vi "Bsweep_VgDep.vi"(5 "Time Stamp":timestamp, 6 "Play Button":bool, 7 "Rate w/o measure, T/min":dbl=0.5 min=0.0 max=1.0 step=0.01 format="%.4f", 9 "Sweep rate, T/min":dbl=0.2 min=0.0 max=1.0 step=0.01 format="%.4f", 10 "B2 (T)":dbl=0.5 min=-4.0 max=4.0 step=0.1 format="%.4f", 11 "B1 (T)":dbl=-0.5 min=-4.0 max=4.0 step=0.1 format="%.4f") -> ()   [LabVIEW 2015]
uses:
  <vilib>/Utility/file.llb/Read From Spreadsheet File (DBL).vi
panel:
  in  "Custom Folder":string
  in  "Hysteresis":bool
  out "VgArray":dbl[](array[numeric])
  in  "Step (V)":dbl=3.0 min=-4.0 max=4.0 step=0.1 format="%.3f"
  in  "Final Vg (V)":dbl=3.0 min=-4.0 max=4.0 step=0.1 format="%.3f"
  in  "Initial Vg (V)":dbl=-3.0 min=-4.0 max=4.0 step=0.1 format="%.3f"
  out "Experiment ends at:":string
  out "Hours":dbl format="%.1f"
  out "Estimated time of experiment:":i16
  in  "Ramp rate (V/min)":dbl=30.0
  in  "Quick Mode":bool=TRUE
  out "Numeric":dbl
  out "Communication":string
  out "ArraySens":i8[](array[numeric])
  out "ArrayOsc":dbl[](array[numeric])
  out "# of configurations":i8
  out "Large Array":bool[][][](array[boolean])
  out "Contact configuration file (*.conf)":path
  # "Set gate voltages at which B-sweeps\nare made"
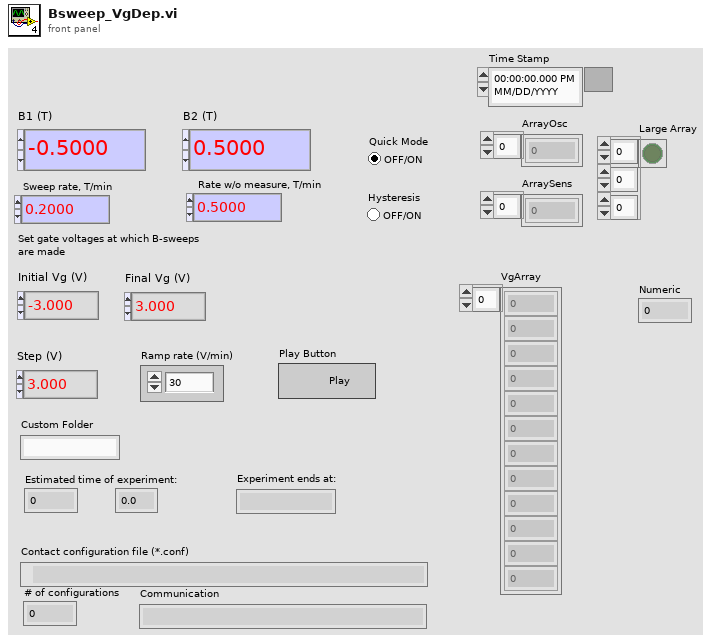
[diagram p1: front panel]
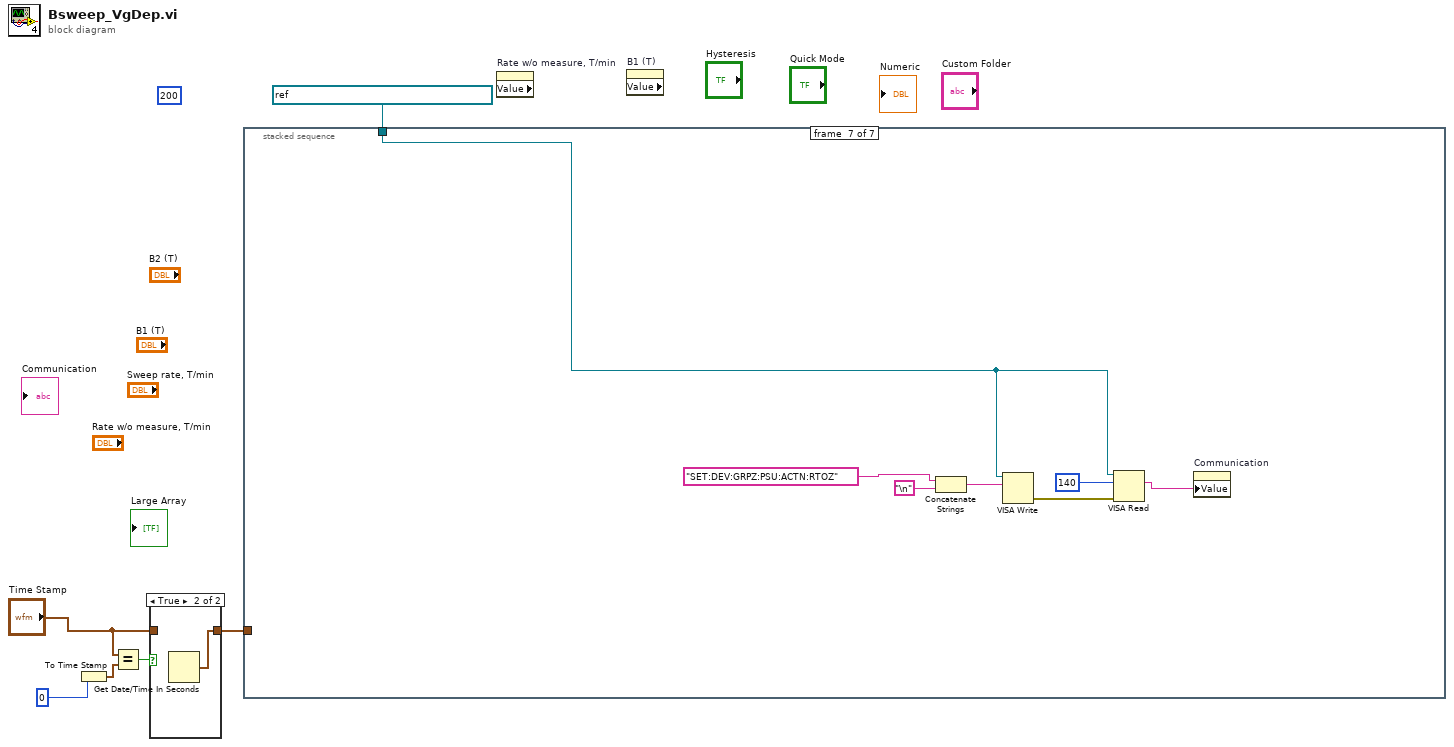
[diagram p0: block diagram]
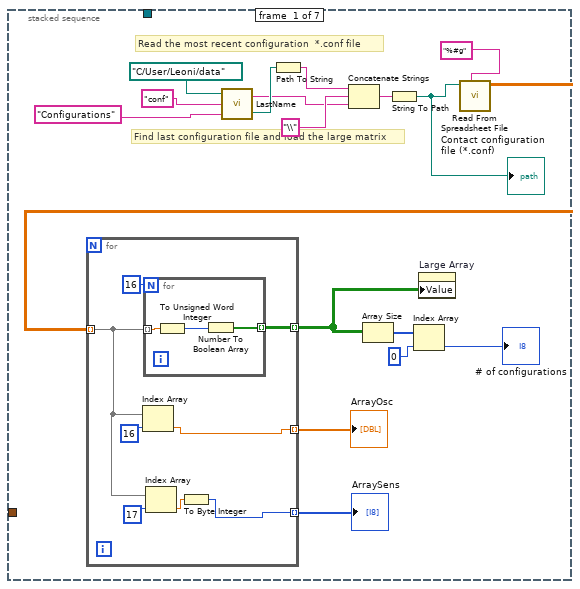
[diagram p3: hidden frame]
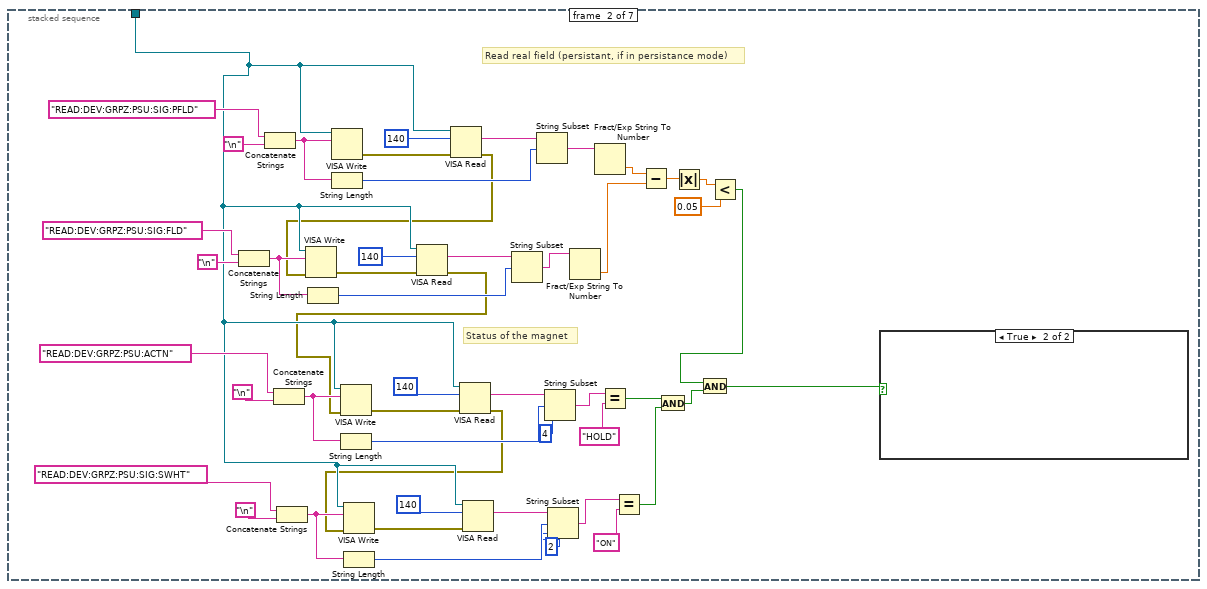
[diagram p4: hidden frame]
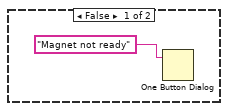
[diagram p5: hidden frame]
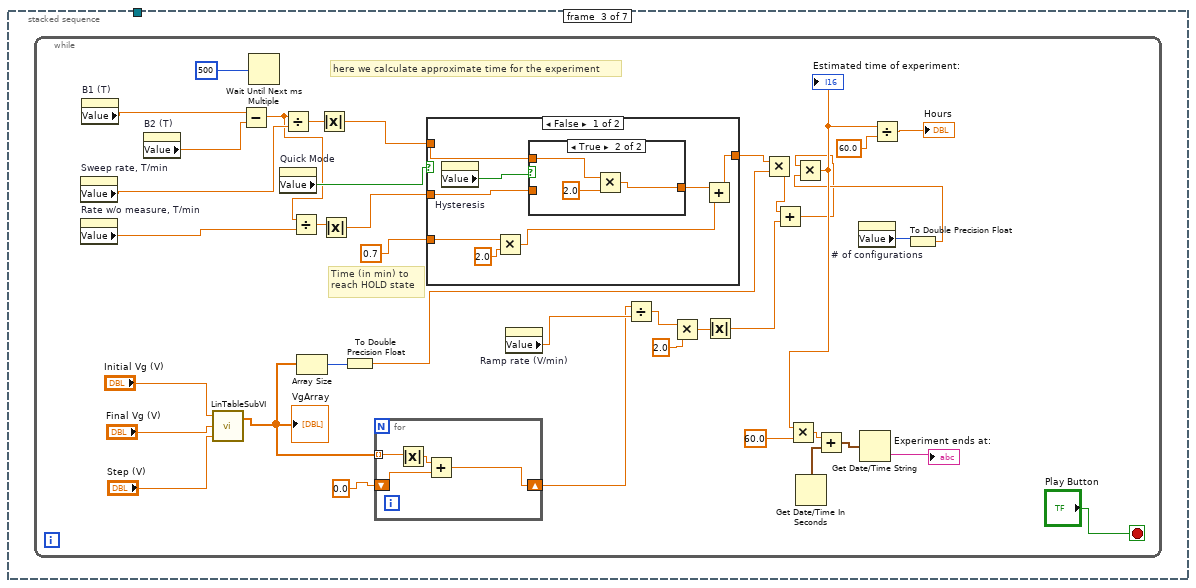
[diagram p6: hidden frame]
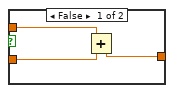
[diagram p7: hidden frame]
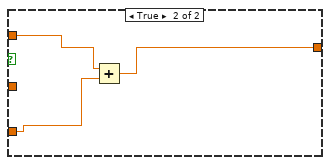
[diagram p8: hidden frame]
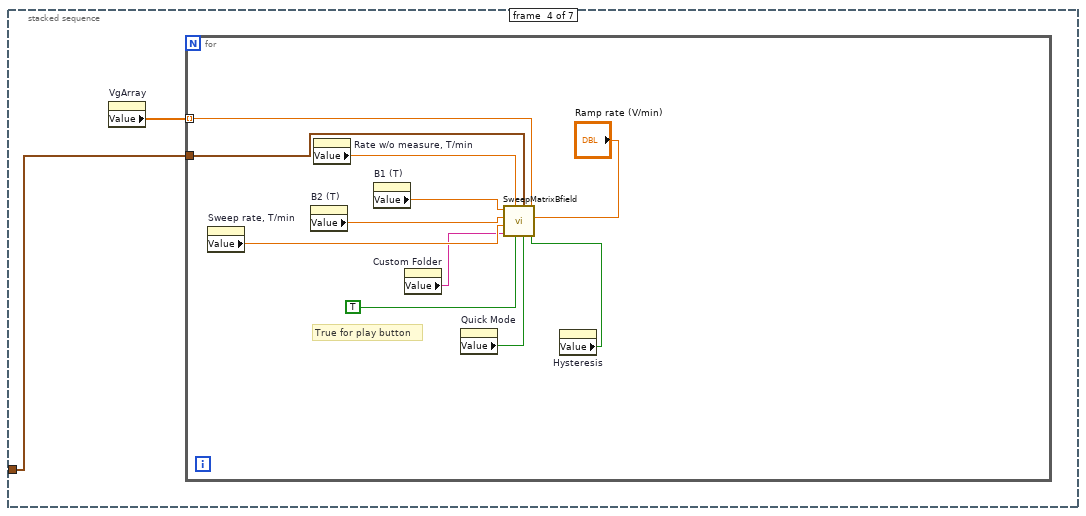
[diagram p9: hidden frame]
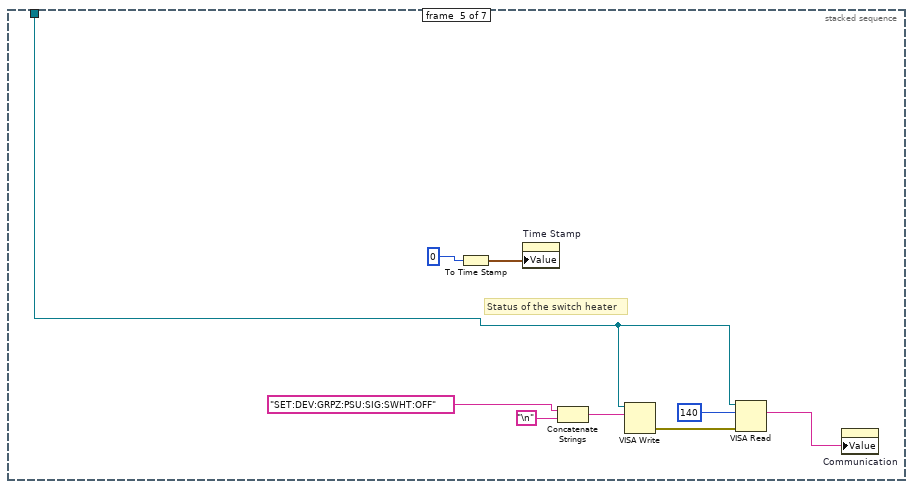
[diagram p10: hidden frame]
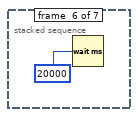
[diagram p11: hidden frame]
diagram:
  (unwired) 200
  n1 = To Time Stamp(1:0) -> (0:w4:timestamp)
  n2 = Equal?(x="Time Stamp", y=w4) -> (x = y?=w3:bool)
  n3 = case shown="True" w3 {
    tunnel: "Time Stamp" -> [w7 _]
    tunnel: [w7 w8] -> w1
    frame False {
    }
    frame True {
      n4 = Get Date/Time In Seconds() -> (seconds since 1Jan1904=w8:timestamp)
    }
  }
  n5 = stacked-sequence {
    tunnel: refnum<visa-resource-name> "TCPIP0::192.168.128.3::7020::SOCKET" ("VISA resource name") -> [_ w40 _ _ w162 _ w172]
    tunnel: w1 -> [_ _ _ w148 _ _ _]
    frame #0 {
      # "Read the most recent configuration  *.conf file"
      # "Find last configuration file and load the large matrix"
      n6 = call "LastName.vi"("Custom Folder"="Configurations", "Extention"="conf", "User Data Folder"=path "C:/User/Leoni/data") -> ("created path"=w21:path, "String"=w20:string)
      n7 = Path To String(path=w21) -> (string=w25:string)
      n8 = Concatenate Strings(w25, "\\", w20) -> (w23:string)
      n9 = String To Path(string=w23) -> (path=w11:path)
      "Contact configuration file (*.conf)" <- w11
      n10 = call-poly <vilib>:"Read From Spreadsheet File.vi"("format (%.3f)"="%#g", "file path (dialog if empty)"=w11) -> ("all rows"=w16:dbl[][])  [unwired: 5 in, 4 out]
      n11 = for {
        tunnel: w16 -> [w29] mode=indexing
        tunnel: [w33] -> w13 mode=indexing
        tunnel: [w28] -> w10 mode=indexing
        tunnel: [w27] -> w9 mode=indexing
        n12 = Index Array(array=w29, index=16) -> (element=w28:dbl)
        n13 = for {
          N: 16 -> [_]
          tunnel: w29 -> [w36] mode=indexing
          tunnel: [w34] -> w33 mode=indexing
          n14 = To Unsigned Word Integer(number=w36) -> (unsigned 16bit integer=w35:u16)
          n15 = Number To Boolean Array(number=w35) -> (Boolean array=w34:bool[])
        }
        n16 = Index Array(array=w29, index=17) -> (element=w30:dbl)
        n17 = To Byte Integer(number=w30) -> (8bit integer=w27:i8)
      }
      "ArrayOsc" <- w10
      "ArraySens" <- w9
      n18 = Array Size(array=w13) -> (size(s)=w15:i32[])
      n19 = Index Array(array=w15, index=0) -> (element=→"# of configurations":i32)
      n20 = property on="Large Array" class="Arr (strict)"("Value"=w13) -> ()  [unwired: 2 in, 2 out]
    }
    frame #1 {
      # "Status of the magnet"
      # "Read real field (persistant, if in persistance mode)"
      n21 = Concatenate Strings("READ:DEV:GRPZ:PSU:SIG:FLD" ("string"), "\n") -> (w74:string)
      n22 = Concatenate Strings("READ:DEV:GRPZ:PSU:SIG:PFLD" ("string"), "\n") -> (w80:string)
      n23 = Concatenate Strings("READ:DEV:GRPZ:PSU:ACTN" ("string"), "\n") -> (w59:string)
      n24 = Concatenate Strings("READ:DEV:GRPZ:PSU:SIG:SWHT" ("string"), "\n") -> (w49:string)
      n25 = String Length(string=w74) -> (length=w72:i32)
      n26 = VISA Write(VISA resource name=w40, write buffer=w80) -> (error out=w86:errorcluster)  [unwired: 1 in, 2 out]
      n27 = String Length(string=w80) -> (length=w81:i32)
      n28 = String Length(string=w59) -> (length=w60:i32)
      n29 = String Length(string=w49) -> (length=w50:i32)
      n30 = VISA Read(VISA resource name=w40, byte count=140, error in (no error)=w86) -> (read buffer=w82:string, error out=w39:errorcluster)  [unwired: 2 out]
      n31 = VISA Write(VISA resource name=w40, write buffer=w74, error in (no error)=w39) -> (error out=w78:errorcluster)  [unwired: 2 out]
      n32 = VISA Read(VISA resource name=w40, byte count=140, error in (no error)=w78) -> (read buffer=w73:string, error out=w38:errorcluster)  [unwired: 2 out]
      n33 = VISA Write(VISA resource name=w40, write buffer=w59, error in (no error)=w38) -> (error out=w65:errorcluster)  [unwired: 2 out]
      n34 = VISA Read(VISA resource name=w40, byte count=140, error in (no error)=w65) -> (read buffer=w61:string, error out=w37:errorcluster)  [unwired: 2 out]
      n35 = VISA Write(VISA resource name=w40, write buffer=w49, error in (no error)=w37) -> (error out=w55:errorcluster)  [unwired: 2 out]
      n36 = VISA Read(VISA resource name=w40, byte count=140, error in (no error)=w55) -> (read buffer=w51:string)  [unwired: 3 out]
      n37 = String Subset(string=w73, offset (0)=w72) -> (substring=w71:string)  [unwired: 1 in]
      n38 = String Subset(string=w82, offset (0)=w81) -> (substring=w79:string)  [unwired: 1 in]
      n39 = String Subset(string=w61, offset (0)=w60, length (rest)=4) -> (substring=w57:string)
      n40 = String Subset(string=w51, offset (0)=w50, length (rest)=2) -> (substring=w46:string)
      n41 = Fract/Exp String To Number(string=w71) -> (number=w69:dbl)  [unwired: 3 in, 1 out]
      n42 = Fract/Exp String To Number(string=w79) -> (number=w70:dbl)  [unwired: 3 in, 1 out]
      n43 = Equal?(x=w57, y="HOLD") -> (x = y?=w45:bool)
      n44 = Equal?(x=w46, y="ON") -> (x = y?=w44:bool)
      n45 = Subtract(x=w70, y=w69) -> (x-y=w68:dbl)
      n46 = And(x=w45, y=w44) -> (x .and. y?=w43:bool)
      n47 = Absolute Value(x=w68) -> (abs(x)=w67:dbl)
      n48 = Less?(x=w67, y=0.05) -> (x < y?=w42:bool)
      n49 = And(x=w42, y=w43) -> (x .and. y?=w41:bool)
      n50 = case shown="True" w41 {
        frame False {
          n51 = One Button Dialog(message="Magnet not ready") -> ()  [unwired: 1 in, 1 out]
        }
        frame True {
        }
      }
    }
    frame #2 {
      n52 = while {
        stop <- "Play Button" stop-if-true
        # "Time (in min) to\nreach HOLD state"
        # "here we calculate approximate time for the experiment"
        n53 = property on="Sweep rate, T/min" class="DigNum (strict)"() -> ("Value"=w112:dbl)  [unwired: 2 in, 2 out]
        n54 = property on="Rate w/o measure, T/min" class="DigNum (strict)"() -> ("Value"=w111:dbl)  [unwired: 2 in, 2 out]
        n55 = property on="B1 (T)" class="DigNum (strict)"() -> ("Value"=w114:dbl)  [unwired: 2 in, 2 out]
        n56 = property on="B2 (T)" class="DigNum (strict)"() -> ("Value"=w113:dbl)  [unwired: 2 in, 2 out]
        n57 = call "LinTableSubVI.vi"("Step"="Step (V)", "Final"="Final Vg (V)", "Initial"="Initial Vg (V)") -> ("Array"=w93:dbl[])  [unwired: 1 in]
        "VgArray" <- w93
        n58 = Subtract(x=w114, y=w113) -> (x-y=w109:dbl)
        n59 = Wait Until Next ms Multiple(millisecond multiple=500) -> ()  [unwired: 1 out]
        n60 = property on="Quick Mode" class="Bool (strict)"() -> ("Value"=w110:bool)  [unwired: 2 in, 2 out]
        n61 = Divide(x=w109, y=w112) -> (x/y=w125:dbl)
        n62 = Divide(x=w109, y=w111) -> (x/y=w100:dbl)
        n63 = Array Size(array=w93) -> (size(s)=w92:i32)
        n64 = Absolute Value(x=w125) -> (abs(x)=w115:dbl)
        n65 = Absolute Value(x=w100) -> (abs(x)=w99:dbl)
        n66 = To Double Precision Float(number=w92) -> (double precision float=w91:dbl)
        n67 = for {
          tunnel: w93 -> [w130] mode=indexing
          shift-right: [w127] -> w94
          shift-left: 0.0 -> [w128]
          n68 = Absolute Value(x=w130) -> (abs(x)=w129:dbl)
          n69 = Add(x=w129, y=w128) -> (x+y=w127:dbl)
        }
        n70 = case shown="False" w110 {
          tunnel: [w132 w145] -> w101
          tunnel: w99 -> [w138 _]
          tunnel: w115 -> [w137 w147]
          tunnel: 0.7 -> [w135 w146]
          frame False {
            n71 = property on="Hysteresis" class="Bool (strict)"() -> ("Value"=w131:bool)  [unwired: 2 in, 2 out]
            n72 = Multiply(x=w135, y=2.0) -> (x*y=w134:dbl)
            n73 = case shown="True" w131 {
              tunnel: w138 -> [w141 _]
              tunnel: w137 -> [w140 w143]
              tunnel: [w139 w142] -> w133
              frame False {
                n74 = Add(x=w140, y=w141) -> (x+y=w139:dbl)
              }
              frame True {
                n75 = Multiply(x=w143, y=2.0) -> (x*y=w142:dbl)
              }
            }
            n76 = Add(x=w133, y=w134) -> (x+y=w132:dbl)
          }
          frame True {
            n77 = Add(x=w147, y=w146) -> (x+y=w145:dbl)
          }
        }
        n78 = property on="Ramp rate (V/min)" class="DigNum (strict)"() -> ("Value"=w104:dbl)  [unwired: 2 in, 2 out]
        n79 = Divide(x=w94, y=w104) -> (x/y=w107:dbl)
        n80 = Multiply(x=w107, y=2.0) -> (x*y=w106:dbl)
        n81 = Absolute Value(x=w106) -> (abs(x)=w89:dbl)
        n82 = Multiply(x=w101, y=w91) -> (x*y=w90:dbl)
        n83 = Add(x=w90, y=w89) -> (x+y=w88:dbl)
        n84 = Get Date/Time In Seconds() -> (seconds since 1Jan1904=w119:timestamp)
        n85 = property on="# of configurations" class="DigNum (strict)"() -> ("Value"=w103:i8)  [unwired: 2 in, 2 out]
        n86 = To Double Precision Float(number=w103) -> (double precision float=w102:dbl)
        n87 = Multiply(x=w88, y=w102) -> (x*y=w116:dbl)
        "Estimated time of experiment:" <- w116
        n88 = Multiply(x=w116, y=60.0) -> (x*y=w120:dbl)
        n89 = Add(x=w120, y=w119) -> (x+y=w118:timestamp)
        n90 = Get Date/Time String(seconds (now)=w118) -> (time string=→"Experiment ends at:":string)  [unwired: 2 in, 1 out]
        n91 = Divide(x=w116, y=60.0) -> (x/y=→"Hours":dbl)
      }
    }
    frame #3 {
      n92 = property on="VgArray" class="Arr (strict)"() -> ("Value"=w149:dbl[])  [unwired: 2 in, 2 out]
      n93 = for {
        tunnel: w149 -> [w160] mode=indexing
        tunnel: w148 -> [w155]
        # "True for play button"
        n94 = property on="Sweep rate, T/min" class="DigNum (strict)"() -> ("Value"=w157:dbl)  [unwired: 2 in, 2 out]
        n95 = property on="B2 (T)" class="DigNum (strict)"() -> ("Value"=w158:dbl)  [unwired: 2 in, 2 out]
        n96 = property on="Rate w/o measure, T/min" class="DigNum (strict)"() -> ("Value"=w156:dbl)  [unwired: 2 in, 2 out]
        n97 = property on="B1 (T)" class="DigNum (strict)"() -> ("Value"=w159:dbl)  [unwired: 2 in, 2 out]
        n98 = property on="Custom Folder" class="Str"() -> ("Value"=w152:string)  [unwired: 2 in, 2 out]
        n99 = property on="Quick Mode" class="Bool (strict)"() -> ("Value"=w154:bool)  [unwired: 2 in, 2 out]
        n100 = property on="Hysteresis" class="Bool (strict)"() -> ("Value"=w153:bool)  [unwired: 2 in, 2 out]
        n101 = call "SweepMatrixBfield.vi"("From B2 to B1"=w153, "Voltage rate (V/min)"="Ramp rate (V/min)", "Voltage (sourse)"=w160, "Change contacts B2 to B1"=w154, "Time Stamp"=w155, "Play Button"=TRUE, "Rate w/o measure, T/min"=w156, "Custom Folder"=w152, "Sweep rate, T/min"=w157, "B2 (T)"=w158, "B1 (T)"=w159) -> ()  [unwired: 1 in]
      }
    }
    frame #4 {
      # "Status of the switch heater"
      n102 = To Time Stamp(1:0) -> (0:w168:timestamp)
      n103 = property on="Time Stamp" class="AbsTime (strict)"("Value"=w168) -> ()  [unwired: 2 in, 2 out]
      n104 = Concatenate Strings("SET:DEV:GRPZ:PSU:SIG:SWHT:OFF" ("string"), "\n") -> (w164:string)
      n105 = VISA Write(VISA resource name=w162, write buffer=w164) -> (error out=w167:errorcluster)  [unwired: 1 in, 2 out]
      n106 = VISA Read(VISA resource name=w162, byte count=140, error in (no error)=w167) -> (read buffer=w161:string)  [unwired: 3 out]
      n107 = property on="Communication" class="Str"("Value"=w161) -> ()  [unwired: 2 in, 2 out]
    }
    frame #5 {
      n108 = Wait (ms)(milliseconds to wait=20000) -> ()  [unwired: 1 out]
    }
    frame #6 {
      n109 = Concatenate Strings("SET:DEV:GRPZ:PSU:ACTN:RTOZ" ("string"), "\n") -> (w174:string)
      n110 = VISA Write(VISA resource name=w172, write buffer=w174) -> (error out=w177:errorcluster)  [unwired: 1 in, 2 out]
      n111 = VISA Read(VISA resource name=w172, byte count=140, error in (no error)=w177) -> (read buffer=w171:string)  [unwired: 3 out]
      n112 = property on="Communication" class="Str"("Value"=w171) -> ()  [unwired: 2 in, 2 out]
    }
  }
  n113 = property on="Rate w/o measure, T/min" class="DigNum (strict)" props=["Value"]() -> ()  [unwired: 2 in, 3 out]
  n114 = property on="B1 (T)" class="DigNum (strict)" props=["Value"]() -> ()  [unwired: 2 in, 3 out]
